vi "Esc Sequence Parser.vi"(11 "read buffer":string) -> (3 "Array":string[][](array[string]))   [LabVIEW 2018]
doc: "This SubVI taskes in a data stream formated in the ANSI Escape sequence code used by a VT100 terminal.\nFrom the Escape code, it retreaves the data along with its relative position (x,y coordinates) on the screen.\nThis information is converted into a 2D array.\nThe format is as follows:\nRow, Column, Data\nWhere row, colunm, and data are 1D arrays."
uses:
  <vilib>/regexp/Match Regular Expression.xnode
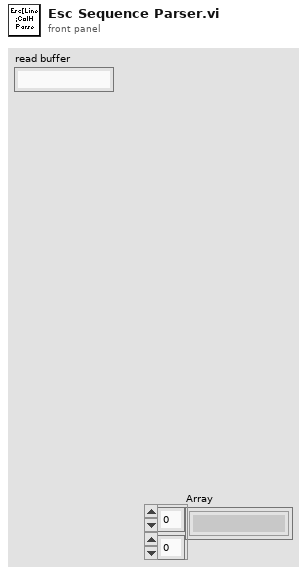
[diagram p1: front panel]
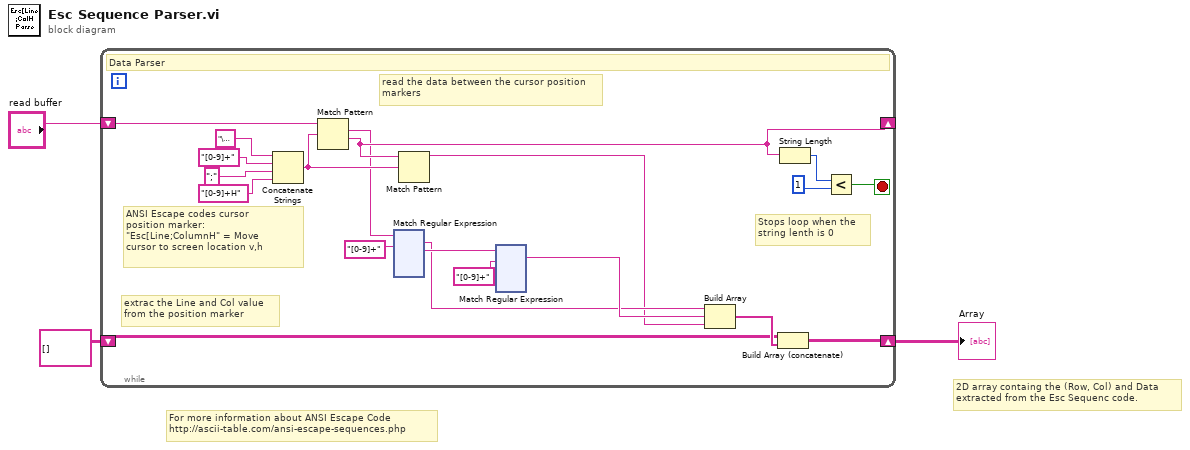
[diagram p0: block diagram]
diagram:
  # "2D array containg the (Row, Col) and Data \nextracted from the Esc Sequenc code."
  # "For more information about ANSI Escape Code\nhttp://ascii-table.com/ansi-escape-sequences.php"
  n1 = while {
    shift-right: [w15] -> _
    shift-left: "read buffer" -> [w23]
    shift-right: [w13] -> w2
    shift-left: string[][] [] -> [w5]
    stop <- w19 stop-if-true
    # "ANSI Escape codes cursor \nposition marker:\n\"Esc[Line;ColumnH\" = Move \ncursor to screen location v,h"
    # "extrac the Line and Col value \nfrom the position marker"
    # "read the data between the cursor position\nmarkers"
    # "Stops loop when the \nstring lenth is 0"
    # "Data Parser"
    n2 = Concatenate Strings("\u001b[" ("string"), "[0-9]+" ("string"), ";" ("string"), "[0-9]+H" ("string")) -> (w14:string)
    n3 = Match Pattern(string=w23, regular expression=w14) -> (match substring=w12:string, after substring=w15:string)  [unwired: 1 in, 2 out]
    n4 = xnode "Match Regular Expression"("input string"=w12, "regular expression"="[0-9]+") -> ("whole match"=w7:string, "after match"=w10:string)  [unwired: 4 in, 4 out]
    n5 = Match Pattern(string=w15, regular expression=w14) -> (before substring=w4:string)  [unwired: 1 in, 3 out]
    n6 = xnode "Match Regular Expression"("input string"=w10, "regular expression"="[0-9]+") -> ("whole match"=w8:string)  [unwired: 4 in, 5 out]
    n7 = Build Array(w7, w8, w4) -> (w6:string[])
    n8 = Build Array (concatenate)(w5, w6) -> (w13:string[][])
    n9 = String Length(string=w15) -> (length=w21:i32)
    n10 = Less?(x=w21, y=1) -> (x < y?=w19:bool)
  }
  "Array" <- w2
